vi "Positioner.vi"(8 "error in (no error)":errorcluster, 10 "Notifiers":T1, 11 "All Message Queue Cluster":T2) -> (0 "error out":errorcluster)   [LabVIEW 2013]
doc: "Ce VI est la partie visualisation du Positioner. Elle permet l'envoie d'ordre à cette appareil et affiche son état.\n- Connected : indique si l'appareil est connecté.\n- Position : indique la postion en mm du positioner.\n- Status : indique le status actuel du positioner. CAD s'il y a une erreur, ou s'il est en mouvement, etc ..."
uses:
  Lib QMH/AllMessageQueue Cluster.ctl
  Lib QMH/Message Cluster.ctl
  Lib Notifier/Notifier.ctl
  Pos UI data.ctl
  Pos Config.ctl
  FGV/Action Pos.ctl
  FGV/FGV Pos Data.ctl
  Lib IHM Control/Front Panel Status.ctl
  support/Status.vi
  Lib QMH/MessageQueues.lvlib
  Lib IHM Control/IHM Control.lvlib
  Lib Notifier/Notifier.lvlib
panel:
  out "Connected":bool
  out "Status":string
  out "Position (mm)":dbl format="%#_3g"
  # "Positionner"
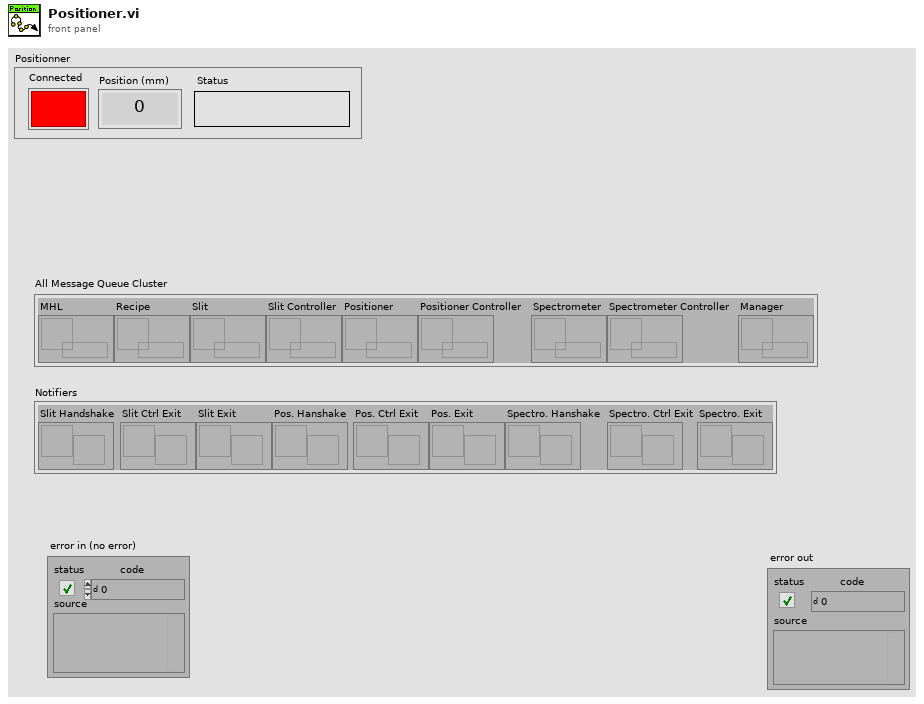
[diagram p1: front panel]
types:
  T1 = typedef "Notifier.lvlib/Notifier.ctl" = cluster{"Slit Handshake":refnum<notifier>, "Slit Ctrl Exit":refnum<notifier>, "Slit Exit":refnum<notifier>, "Pos. Hanshake":refnum<notifier>, "Pos. Ctrl Exit":refnum<notifier>, "Pos. Exit":refnum<notifier>, "Spectro. Hanshake":refnum<notifier>, "Spectro. Ctrl Exit":refnum<notifier>, "Spectro. Exit":refnum<notifier>}
  T2 = typedef "MessageQueues.lvlib/AllMessageQueue Cluster.ctl" = cluster{"MHL":refnum<queue>, "Recipe":refnum<queue>, "Slit":refnum<queue>, "Slit Controller":refnum<queue>, "Positioner":refnum<queue>, "Positioner Controller":refnum<queue>, "Spectrometer":refnum<queue>, "Spectrometer Controller":refnum<queue>, "Manager":refnum<queue>}
  T3 = typedef "Pos Config.ctl" = cluster{"VISA resource name":refnum<visa-resource-name>}
  T4 = typedef "Pos UI data.ctl" = cluster{"Connected":bool, "Status":string, "Position":dbl}
  T5 = typedef "Action Pos.ctl" = enum16{"Connect", "Initialize", "Set Velocity", "Get Velocity", "Move Rel", "Move Abs", "Position", "Status", "Abort", "Disconnect"}
  T6 = typedef "FGV Pos Data.ctl" = cluster{"Portnumber":i32, "Position":dbl, "Status":string, "Système ID":i32, "Connected axes":string[], "Velocity":dbl, "Stage names":string[], "Device ID out":i32}
  T7 = typedef "IHM Control.lvlib/Front Panel Status.ctl" = enum16{"Initialisation", "Enable Slit", "Enable Positionner", "Enable Spectrometer", "Disable Slit", "Disable Positionner", "Disable Spectrometer"}
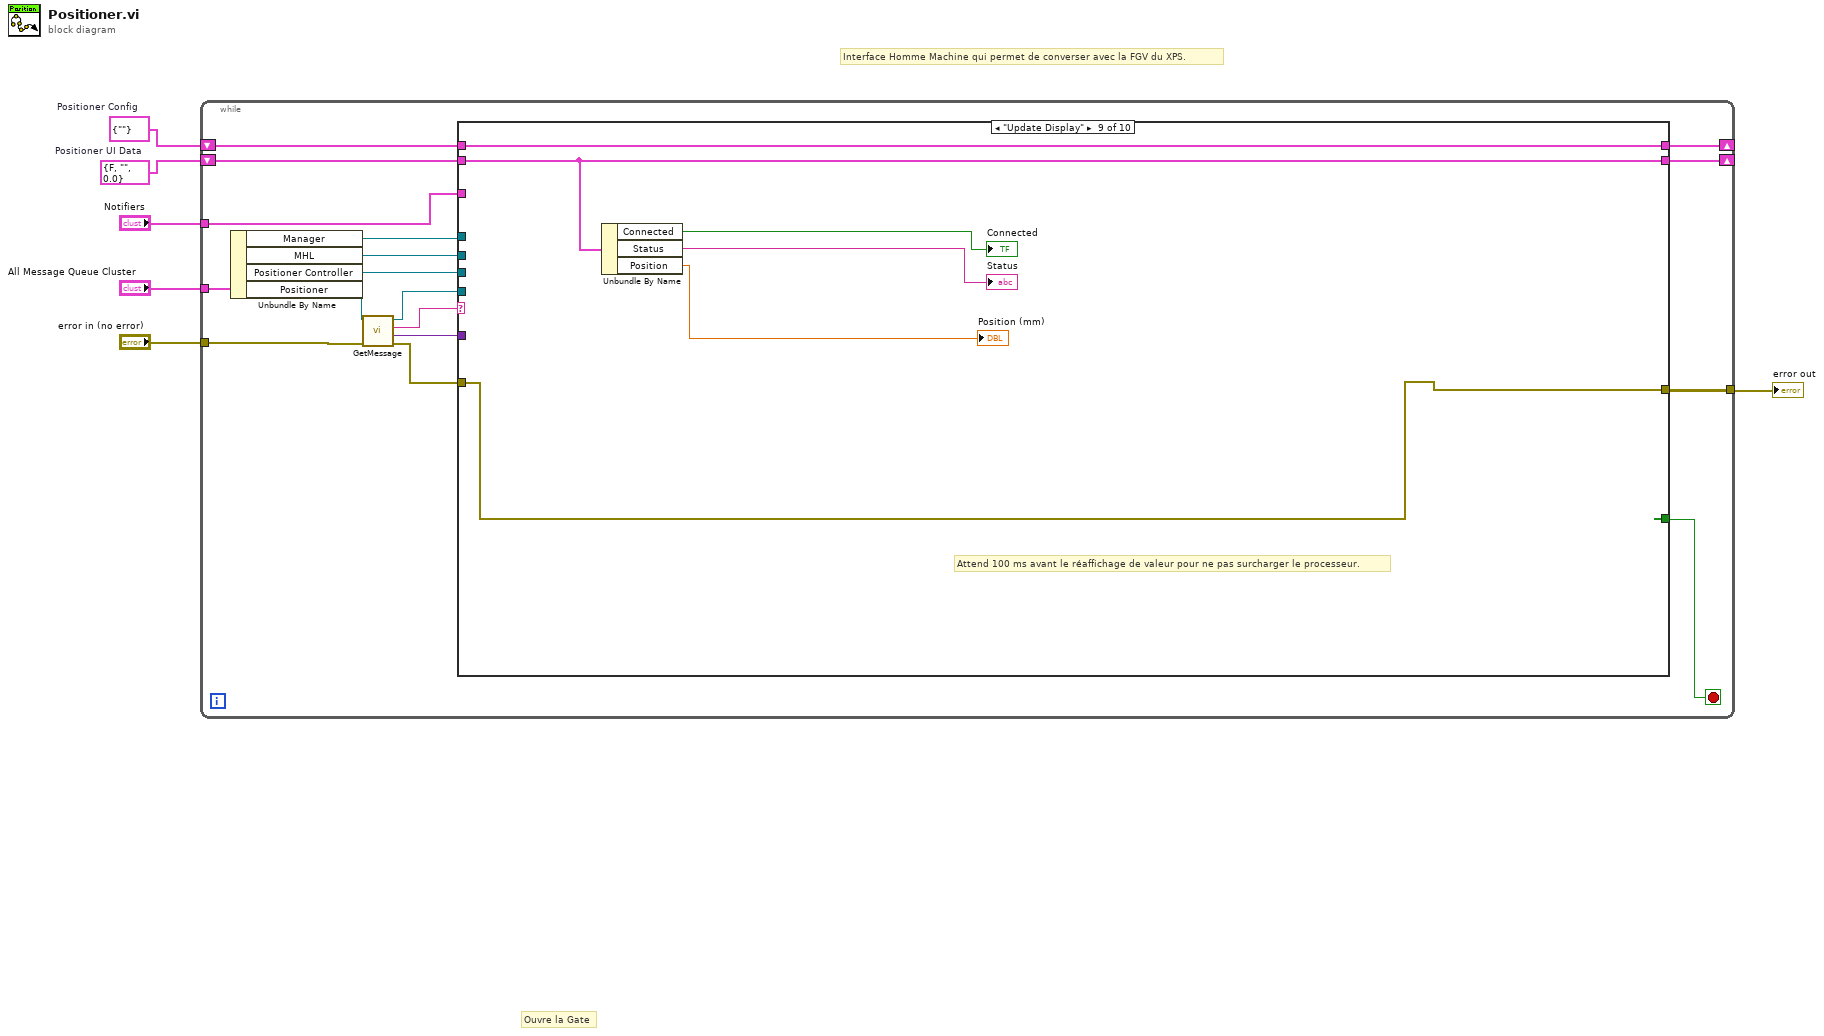
[diagram p0: block diagram]
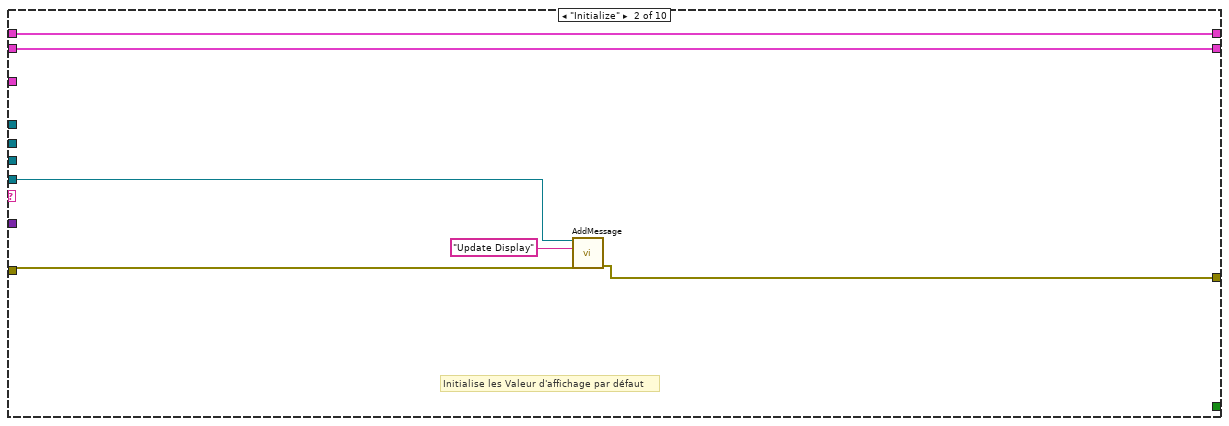
[diagram p3: hidden frame]
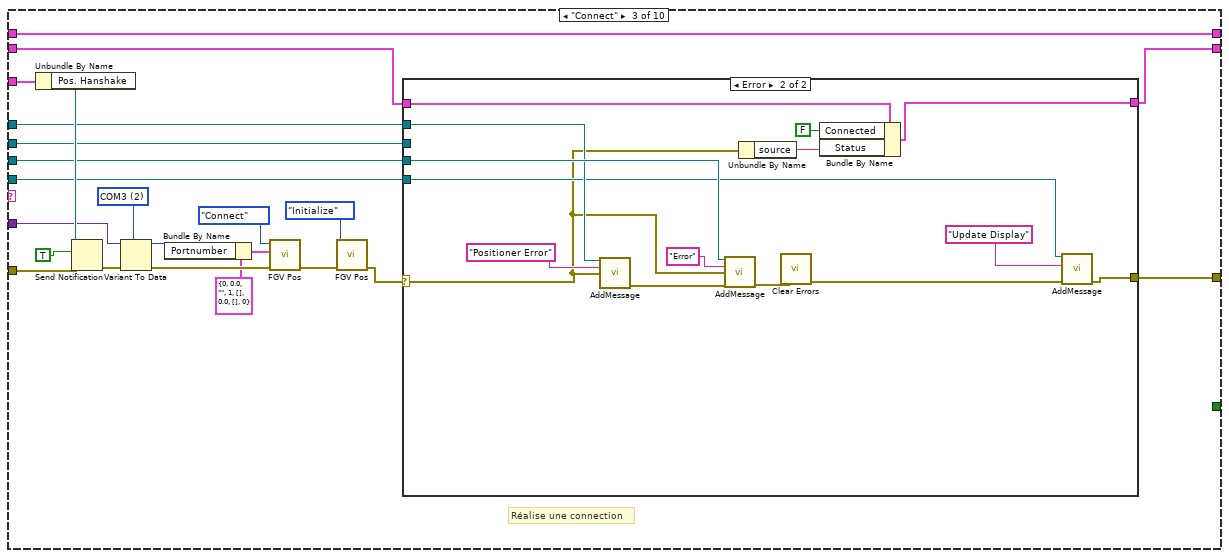
[diagram p4: hidden frame]
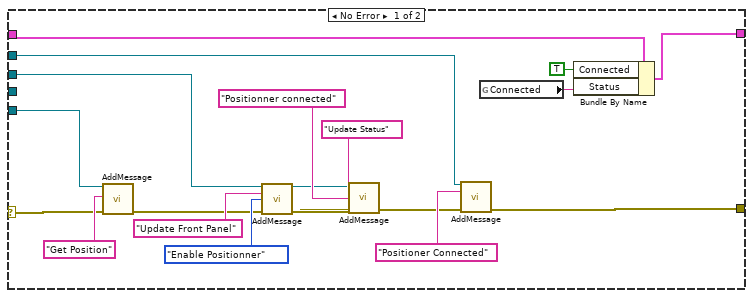
[diagram p5: hidden frame]
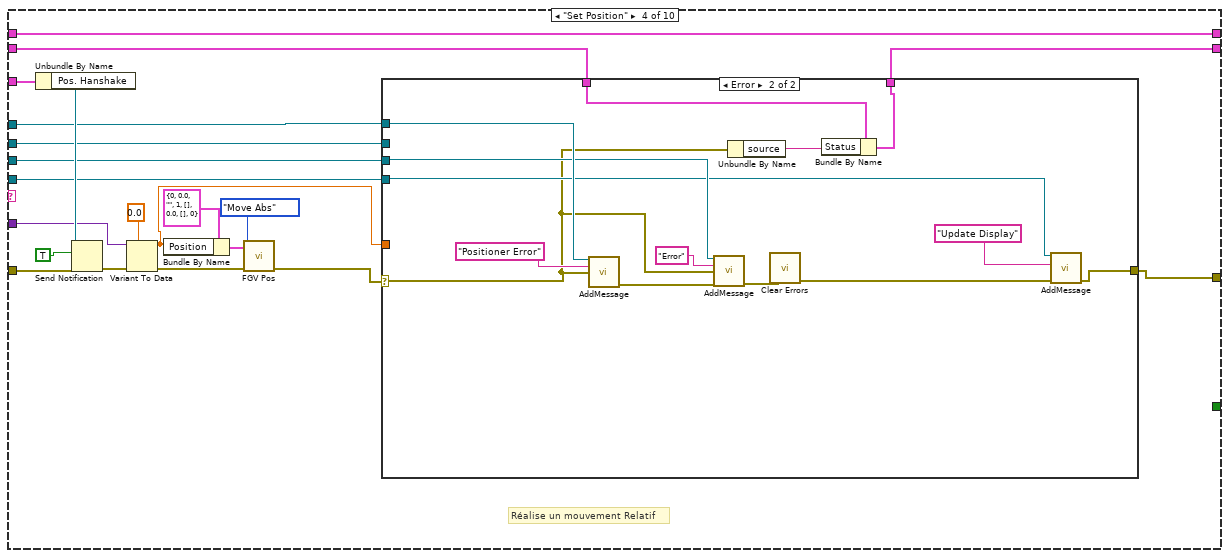
[diagram p6: hidden frame]
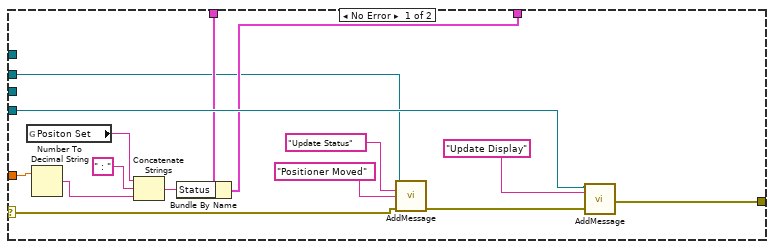
[diagram p7: hidden frame]
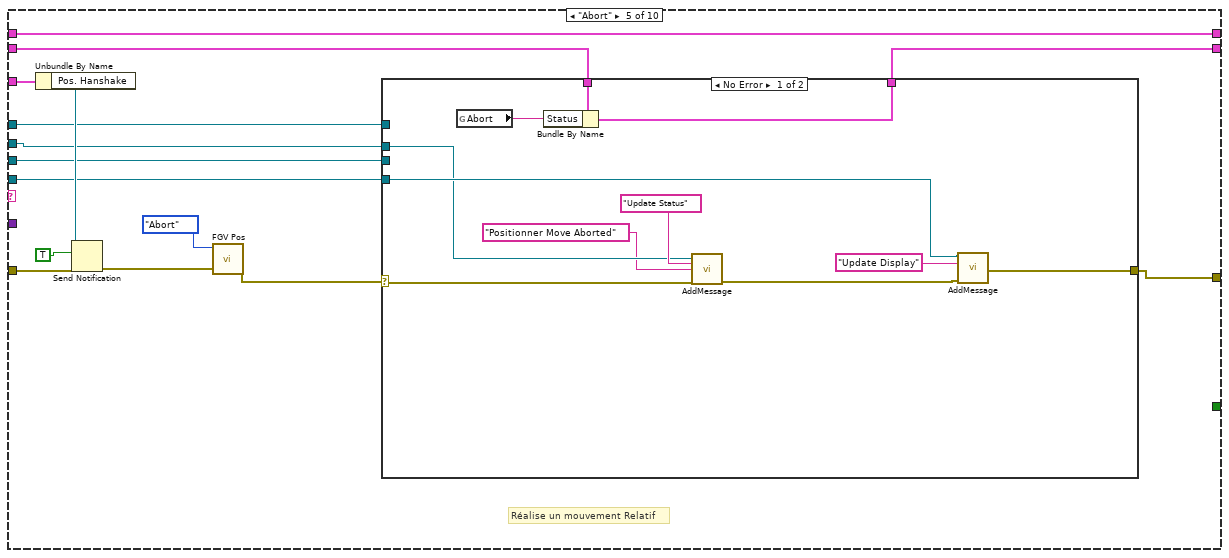
[diagram p8: hidden frame]
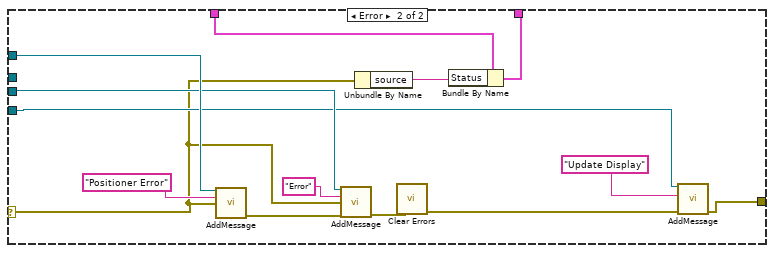
[diagram p9: hidden frame]
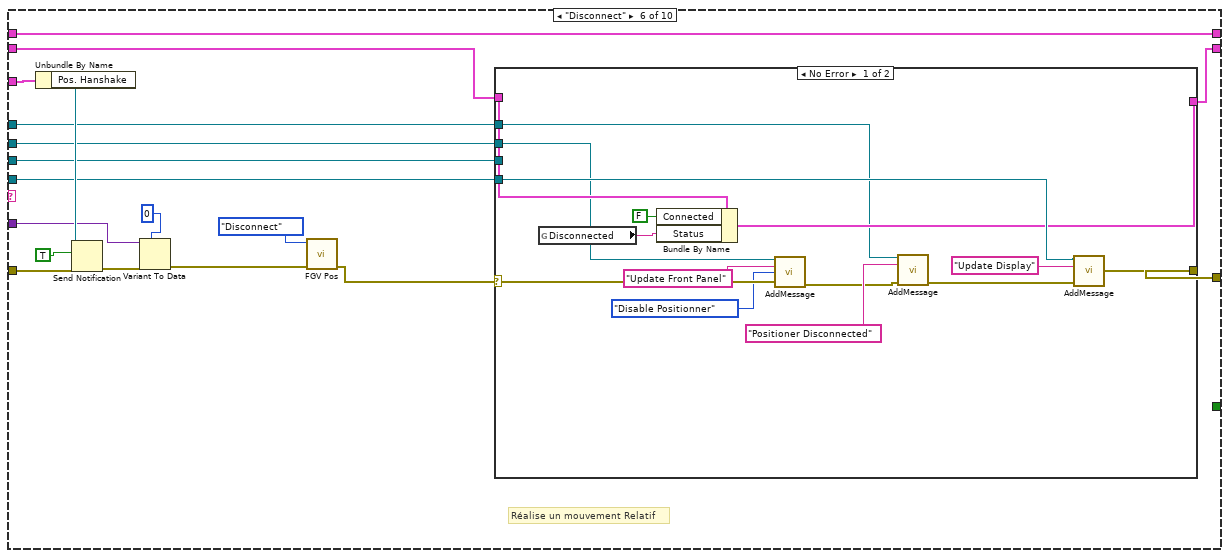
[diagram p10: hidden frame]
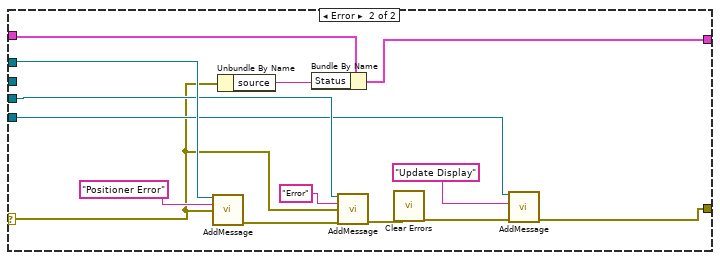
[diagram p11: hidden frame]
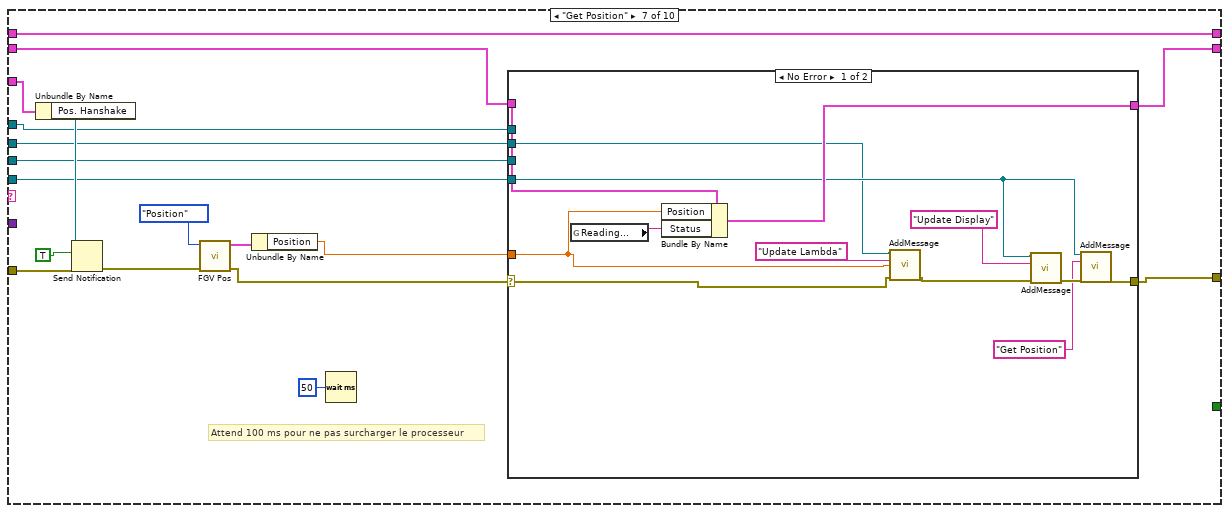
[diagram p12: hidden frame]
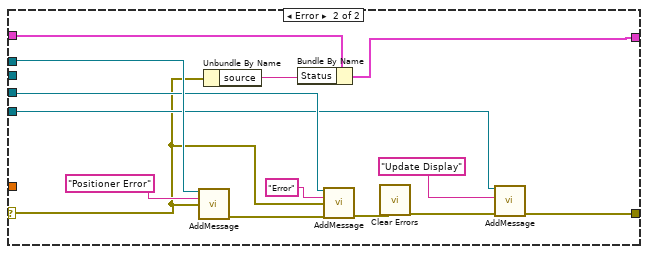
[diagram p13: hidden frame]
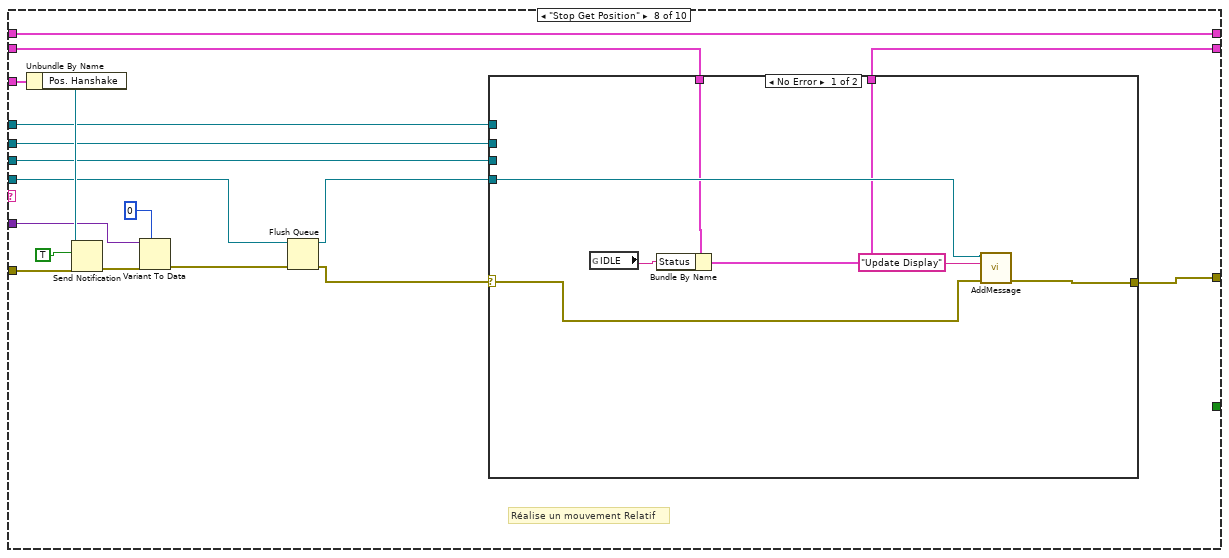
[diagram p14: hidden frame]
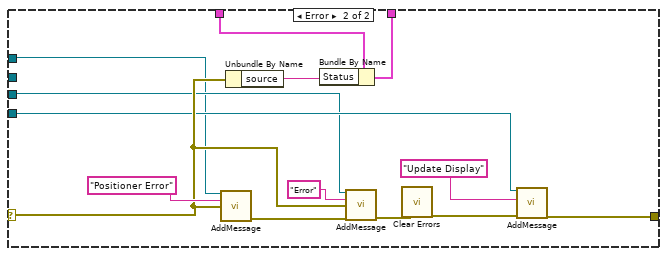
[diagram p15: hidden frame]
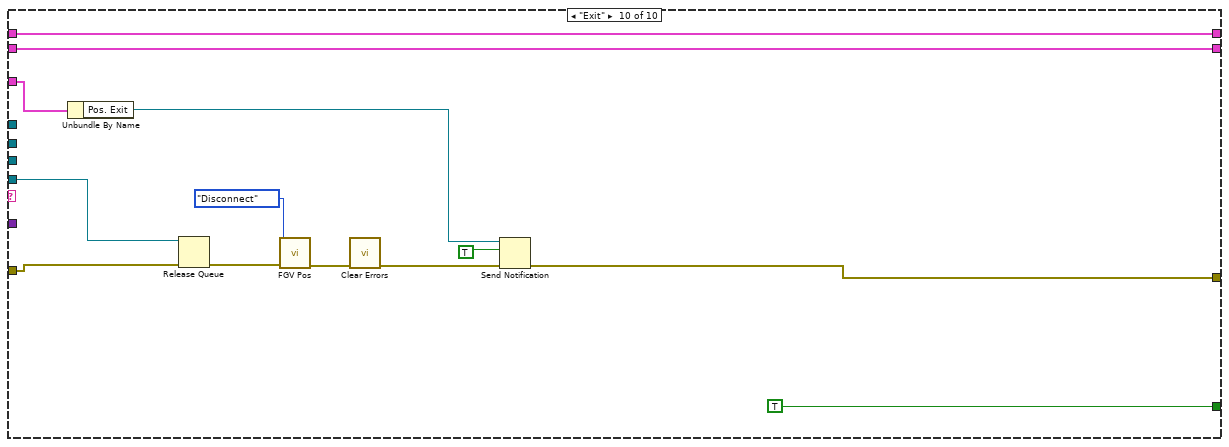
[diagram p16: hidden frame]
diagram:
  w1 = T3 {"VISA resource name"=""}  # Positioner Config
  w2 = T4 {"Connected"=FALSE, "Status"="", "Position"=0.0}  # Positioner UI Data
  # "Interface Homme Machine qui permet de converser avec la FGV du XPS."
  # "Ouvre la Gate"
  n1 = while {
    tunnel: "All Message Queue Cluster" -> [w21]
    tunnel: "Notifiers" -> [w18]
    tunnel: "error in (no error)" -> [w22]
    tunnel: [w10] -> w3
    shift-right: [w8] -> _
    shift-left: w1 -> [w20]
    shift-right: [w9] -> _
    shift-left: w2 -> [w19]
    stop <- w7 stop-if-true
    n2 = Unbundle By Name(w21) -> ("Manager"=w11:refnum<queue>, "MHL"=w12:refnum<queue>, "Positioner Controller"=w13:refnum<queue>, "Positioner"=w23:refnum<queue>)
    n3 = call "GetMessage.vi"("entrée d'erreur"=w22, "Message queue"=w23) -> ("sortie d'erreur"=w17:errorcluster, "Data"=w16:variant, "Message"=w15:string, "Dup Message Queue"=w14:refnum<queue>)  [unwired: 6 in]
    n4 = case shown="\"Update Display\"" w15 {
      tunnel: w18 -> [_ _ w53 w108 w152 w195 w242 w287 _ w328]
      tunnel: w14 -> [_ w27 w52 w107 w151 w194 w241 w275 _ w322]
      tunnel: w16 -> [_ _ w41 w97 _ w186 _ w279 _ _]
      tunnel: w17 -> [w26 w30 w46 w101 w145 w188 w236 w281 w315 w323]
      tunnel: [w26 w29 w51 w106 w150 w193 w240 w286 w315 w325] -> w10
      tunnel: w13 -> [_ _ w50 w105 w149 w192 w239 w285 _ _]
      tunnel: [_ _ _ _ _ _ _ _ _ TRUE] -> w7
      tunnel: w20 -> [w25 w32 w49 w104 w148 w191 w238 w284 w316 w324]
      tunnel: [w25 w32 w49 w104 w148 w191 w238 w284 w316 w324] -> w8
      tunnel: w19 -> [w24 w28 w48 w103 w147 w190 w233 w283 w314 w321]
      tunnel: [w24 w28 w47 w102 w146 w189 w237 w282 w314 w321] -> w9
      tunnel: w12 -> [_ _ w45 w100 w144 w184 w234 w272 _ _]
      tunnel: w11 -> [_ _ w44 w99 w143 w183 w227 w273 _ _]
      frame Default {
        # "ne fait rien si le message dépilé n'existe pas"
      }
      frame "Initialize" {
        # "Initialise les Valeur d'affichage par défaut"
        n5 = call "AddMessage.vi"("Message queue"=w27, "Message"="Update Display", "entrée d'erreur (pas d'erreur)"=w30) -> ("error out"=w29:errorcluster)  [unwired: 11 in, 1 out]
      }
      frame "Connect" {
        w42 = 2 items=["COM1", "COM2", "COM3", "COM4", "COM5", "COM6", "COM7", "COM8", "COM9", "COM10", "COM11", "COM12", "COM13", "COM14", "COM15", "COM16", "COM17", "COM18", "COM19", "COM20", "COM21", "COM22", "COM23", "COM24", "COM25", "COM26", "COM27", "COM28", "COM29", "COM30"] ("Portnumber")
        # "Réalise une connection"
        n6 = Unbundle By Name(w53) -> ("Pos. Hanshake"=w55:refnum<notifier>)
        n7 = Send Notification(notification=TRUE, notifier=w55, error in (no error)=w46) -> (error out=w43:errorcluster)  [unwired: 1 out]
        n8 = Variant To Data(error in=w43, type=w42, Variant=w41) -> (data=w37:i32, error out=w40:errorcluster)
        n9 = Bundle By Name(cluster=T6 {"Portnumber"=0, "Position"=0.0, "Status"="", "Système ID"=1, "Connected axes"=[], "Velocity"=0.0, "Stage names"=[], "Device ID out"=0} ("FGV Pos Data"), "Portnumber"=w37) -> (w36:T6)
        n10 = call "FGV Pos.vi"("error in (no error)"=w40, "FGV Pos Data In"=w36, "Action"=Action_Pos."Connect") -> ("error out"=w35:errorcluster)  [unwired: 7 in, 1 out]
        n11 = call "FGV Pos.vi"("error in (no error)"=w35, "Action"=Action_Pos."Initialize") -> ("error out"=w34:errorcluster)  [unwired: 8 in, 1 out]
        n12 = case shown="Error" w34 {
          selector: w34 -> [w59 w76]
          tunnel: w52 -> [w57 w81]
          tunnel: [w61 w85] -> w51
          tunnel: w50 -> [_ w84]
          tunnel: w48 -> [w74 w80]
          tunnel: [w73 w79] -> w47
          tunnel: w45 -> [w71 _]
          tunnel: w44 -> [w66 w82]
          frame No Error {
            n13 = call "AddMessage.vi"("Message queue"=w57, "Message"="Get Position", "entrée d'erreur (pas d'erreur)"=w59) -> ("error out"=w58:errorcluster)  [unwired: 11 in, 1 out]
            n14 = call "AddMessage.vi"("Message queue"=w71, "Message"="Update Front Panel", "Data"=Front_Panel_Status."Enable Positionner" ("Front Panel status"), "entrée d'erreur (pas d'erreur)"=w58) -> ("Dup Message queue"=w63:refnum<queue>, "error out"=w62:errorcluster)  [unwired: 10 in]
            n15 = call "AddMessage.vi"("Message queue"=w63, "Message"="Update Status", "Data"="Positionner connected" ("Message"), "entrée d'erreur (pas d'erreur)"=w62) -> ("error out"=w56:errorcluster)  [unwired: 10 in, 1 out]
            n16 = call "AddMessage.vi"("Message queue"=w66, "Message"="Positioner Connected", "entrée d'erreur (pas d'erreur)"=w56) -> ("error out"=w61:errorcluster)  [unwired: 11 in, 1 out]
            n17 = global read "Status.vi" "Connected"() -> (w67:string)
            n18 = Bundle By Name(cluster=w74, "Connected"=TRUE, "Status"=w67) -> (w73:T4)
          }
          frame Error {
            n19 = call "AddMessage.vi"("Message queue"=w82, "Message"="Positioner Error", "Data"=w76) -> ("error out"=w75:errorcluster)  [unwired: 11 in, 1 out]
            n20 = call "AddMessage.vi"("Message queue"=w84, "Message"="Error", "Data"=w76, "entrée d'erreur (pas d'erreur)"=w75) -> ("error out"=w88:errorcluster)  [unwired: 10 in, 1 out]
            n21 = Unbundle By Name(w76) -> ("source"=w77:string)
            n22 = call <vilib>:"Clear Errors.vi"("error in (no error)"=w88) -> ("error out"=w86:errorcluster)  [unwired: 6 in]
            n23 = Bundle By Name(cluster=w80, "Connected"=FALSE, "Status"=w77) -> (w79:T4)
            n24 = call "AddMessage.vi"("Message queue"=w81, "Message"="Update Display", "entrée d'erreur (pas d'erreur)"=w86) -> ("error out"=w85:errorcluster)  [unwired: 11 in, 1 out]
          }
        }
      }
      frame "Set Position" {
        # "Réalise un mouvement Relatif"
        n25 = Unbundle By Name(w108) -> ("Pos. Hanshake"=w110:refnum<notifier>)
        n26 = Send Notification(notification=TRUE, notifier=w110, error in (no error)=w101) -> (error out=w98:errorcluster)  [unwired: 1 out]
        n27 = Variant To Data(error in=w98, type=0.0, Variant=w97) -> (data=w90:dbl, error out=w95:errorcluster)
        n28 = Bundle By Name(cluster=T6 {"Portnumber"=0, "Position"=0.0, "Status"="", "Système ID"=1, "Connected axes"=[], "Velocity"=0.0, "Stage names"=[], "Device ID out"=0} ("FGV Pos Data"), "Position"=w90) -> (w92:T6)
        n29 = call "FGV Pos.vi"("error in (no error)"=w95, "FGV Pos Data In"=w92, "Action"=Action_Pos."Move Abs") -> ("error out"=w94:errorcluster)  [unwired: 7 in, 1 out]
        n30 = case shown="Error" w94 {
          selector: w94 -> [w113 w127]
          tunnel: w107 -> [w125 w128]
          tunnel: [w123 w126] -> w106
          tunnel: w105 -> [_ w129]
          tunnel: w103 -> [w122 w132]
          tunnel: [w121 w131] -> w102
          tunnel: w100 -> [w111 _]
          tunnel: w99 -> [_ w130]
          tunnel: w90 -> [w117 _]
          frame No Error {
            n31 = global read "Status.vi" "Positon Set"() -> (w120:string)
            n32 = Number To Decimal String(number=w117) -> (decimal integer string=w116:string)  [unwired: 1 in]
            n33 = Concatenate Strings(w120, " : " ("string"), w116) -> (w119:string)
            n34 = Bundle By Name(cluster=w122, "Status"=w119) -> (w121:T4)
            n35 = call "AddMessage.vi"("Message queue"=w111, "Message"="Update Status", "Data"="Positioner Moved" ("Message"), "entrée d'erreur (pas d'erreur)"=w113) -> ("error out"=w112:errorcluster)  [unwired: 10 in, 1 out]
            n36 = call "AddMessage.vi"("Message queue"=w125, "Message"="Update Display", "entrée d'erreur (pas d'erreur)"=w112) -> ("error out"=w123:errorcluster)  [unwired: 11 in, 1 out]
          }
          frame Error {
            n37 = call "AddMessage.vi"("Message queue"=w130, "Message"="Positioner Error", "Data"=w127) -> ("error out"=w133:errorcluster)  [unwired: 11 in, 1 out]
            n38 = call "AddMessage.vi"("Message queue"=w129, "Message"="Error", "Data"=w127, "entrée d'erreur (pas d'erreur)"=w133) -> ("error out"=w138:errorcluster)  [unwired: 10 in, 1 out]
            n39 = Unbundle By Name(w127) -> ("source"=w134:string)
            n40 = call <vilib>:"Clear Errors.vi"("error in (no error)"=w138) -> ("error out"=w136:errorcluster)  [unwired: 6 in]
            n41 = Bundle By Name(cluster=w132, "Status"=w134) -> (w131:T4)
            n42 = call "AddMessage.vi"("Message queue"=w128, "Message"="Update Display", "entrée d'erreur (pas d'erreur)"=w136) -> ("error out"=w126:errorcluster)  [unwired: 11 in, 1 out]
          }
        }
      }
      frame "Abort" {
        # "Réalise un mouvement Relatif"
        n43 = Unbundle By Name(w152) -> ("Pos. Hanshake"=w154:refnum<notifier>)
        n44 = Send Notification(notification=TRUE, notifier=w154, error in (no error)=w145) -> (error out=w142:errorcluster)  [unwired: 1 out]
        n45 = call "FGV Pos.vi"("error in (no error)"=w142, "Action"=Action_Pos."Abort") -> ("error out"=w141:errorcluster)  [unwired: 8 in, 1 out]
        n46 = case shown="No Error" w141 {
          selector: w141 -> [w158 w169]
          tunnel: w151 -> [w165 w170]
          tunnel: [w163 w166] -> w150
          tunnel: w149 -> [_ w171]
          tunnel: w147 -> [w162 w168]
          tunnel: [w161 w167] -> w146
          tunnel: w144 -> [w157 _]
          tunnel: w143 -> [_ w172]
          frame No Error {
            n47 = global read "Status.vi" "Abort"() -> (w160:string)
            n48 = Bundle By Name(cluster=w162, "Status"=w160) -> (w161:T4)
            n49 = call "AddMessage.vi"("Message queue"=w157, "Message"="Update Status", "Data"="Positionner Move Aborted" ("Message"), "entrée d'erreur (pas d'erreur)"=w158) -> ("error out"=w155:errorcluster)  [unwired: 10 in, 1 out]
            n50 = call "AddMessage.vi"("Message queue"=w165, "Message"="Update Display", "entrée d'erreur (pas d'erreur)"=w155) -> ("error out"=w163:errorcluster)  [unwired: 11 in, 1 out]
          }
          frame Error {
            n51 = call "AddMessage.vi"("Message queue"=w172, "Message"="Positioner Error", "Data"=w169) -> ("error out"=w173:errorcluster)  [unwired: 11 in, 1 out]
            n52 = call "AddMessage.vi"("Message queue"=w171, "Message"="Error", "Data"=w169, "entrée d'erreur (pas d'erreur)"=w173) -> ("error out"=w178:errorcluster)  [unwired: 10 in, 1 out]
            n53 = Unbundle By Name(w169) -> ("source"=w174:string)
            n54 = call <vilib>:"Clear Errors.vi"("error in (no error)"=w178) -> ("error out"=w176:errorcluster)  [unwired: 6 in]
            n55 = Bundle By Name(cluster=w168, "Status"=w174) -> (w167:T4)
            n56 = call "AddMessage.vi"("Message queue"=w170, "Message"="Update Display", "entrée d'erreur (pas d'erreur)"=w176) -> ("error out"=w166:errorcluster)  [unwired: 11 in, 1 out]
          }
        }
      }
      frame "Disconnect" {
        # "Réalise un mouvement Relatif"
        n57 = Unbundle By Name(w195) -> ("Pos. Hanshake"=w197:refnum<notifier>)
        n58 = Send Notification(notification=TRUE, notifier=w197, error in (no error)=w188) -> (error out=w187:errorcluster)  [unwired: 1 out]
        n59 = Variant To Data(error in=w187, type=0, Variant=w186) -> (error out=w182:errorcluster)  [unwired: 1 out]
        n60 = call "FGV Pos.vi"("error in (no error)"=w182, "Action"=Action_Pos."Disconnect") -> ("error out"=w181:errorcluster)  [unwired: 8 in, 1 out]
        n61 = case shown="No Error" w181 {
          selector: w181 -> [w206 w216]
          tunnel: w194 -> [w212 w217]
          tunnel: [w210 w215] -> w193
          tunnel: w192 -> [_ w218]
          tunnel: w190 -> [w209 w214]
          tunnel: [w208 w213] -> w189
          tunnel: w184 -> [w205 _]
          tunnel: w183 -> [w199 w219]
          frame No Error {
            n62 = global read "Status.vi" "Disconnected"() -> (w198:string)
            n63 = Bundle By Name(cluster=w209, "Connected"=FALSE, "Status"=w198) -> (w208:T4)
            n64 = call "AddMessage.vi"("Message queue"=w205, "Message"="Update Front Panel", "Data"=Front_Panel_Status."Disable Positionner" ("Front Panel status"), "entrée d'erreur (pas d'erreur)"=w206) -> ("error out"=w201:errorcluster)  [unwired: 10 in, 1 out]
            n65 = call "AddMessage.vi"("Message queue"=w199, "Message"="Positioner Disconnected", "entrée d'erreur (pas d'erreur)"=w201) -> ("error out"=w200:errorcluster)  [unwired: 11 in, 1 out]
            n66 = call "AddMessage.vi"("Message queue"=w212, "Message"="Update Display", "entrée d'erreur (pas d'erreur)"=w200) -> ("error out"=w210:errorcluster)  [unwired: 11 in, 1 out]
          }
          frame Error {
            n67 = call "AddMessage.vi"("Message queue"=w219, "Message"="Positioner Error", "Data"=w216) -> ("error out"=w220:errorcluster)  [unwired: 11 in, 1 out]
            n68 = Unbundle By Name(w216) -> ("source"=w221:string)
            n69 = Bundle By Name(cluster=w214, "Status"=w221) -> (w213:T4)
            n70 = call "AddMessage.vi"("Message queue"=w218, "Message"="Error", "Data"=w216, "entrée d'erreur (pas d'erreur)"=w220) -> ("error out"=w225:errorcluster)  [unwired: 10 in, 1 out]
            n71 = call <vilib>:"Clear Errors.vi"("error in (no error)"=w225) -> ("error out"=w223:errorcluster)  [unwired: 6 in]
            n72 = call "AddMessage.vi"("Message queue"=w217, "Message"="Update Display", "entrée d'erreur (pas d'erreur)"=w223) -> ("error out"=w215:errorcluster)  [unwired: 11 in, 1 out]
          }
        }
      }
      frame "Get Position" {
        # "Attend 100 ms pour ne pas surcharger le processeur"
        n73 = Unbundle By Name(w242) -> ("Pos. Hanshake"=w244:refnum<notifier>)
        n74 = Send Notification(notification=TRUE, notifier=w244, error in (no error)=w236) -> (error out=w232:errorcluster)  [unwired: 1 out]
        n75 = call "FGV Pos.vi"("error in (no error)"=w232, "Action"=Action_Pos."Position") -> ("error out"=w230:errorcluster, "FGV Pos Data Out"=w229:T6)  [unwired: 8 in]
        n76 = Unbundle By Name(w229) -> ("Position"=w228:dbl)
        n77 = Wait (ms)(milliseconds to wait=u32 50) -> ()  [unwired: 1 out]
        n78 = case shown="No Error" w230 {
          selector: w230 -> [w248 w258]
          tunnel: w241 -> [w252 w259]
          tunnel: [w253 w264] -> w240
          tunnel: w239 -> [_ w260]
          tunnel: w233 -> [w256 w262]
          tunnel: [w255 w263] -> w237
          tunnel: w234 -> [w246 _]
          tunnel: w228 -> [w245 _]
          tunnel: w227 -> [_ w261]
          frame No Error {
            n79 = global read "Status.vi" "Reading..."() -> (w250:string)
            n80 = Bundle By Name(cluster=w256, "Position"=w245, "Status"=w250) -> (w255:T4)
            n81 = call "AddMessage.vi"("Message queue"=w246, "Message"="Update Lambda", "Data"=w245, "entrée d'erreur (pas d'erreur)"=w248) -> ("error out"=w247:errorcluster)  [unwired: 10 in, 1 out]
            n82 = call "AddMessage.vi"("Message queue"=w252, "Message"="Update Display", "entrée d'erreur (pas d'erreur)"=w247) -> ("error out"=w254:errorcluster)  [unwired: 11 in, 1 out]
            n83 = call "AddMessage.vi"("Message queue"=w252, "Message"="Get Position", "entrée d'erreur (pas d'erreur)"=w254) -> ("error out"=w253:errorcluster)  [unwired: 11 in, 1 out]
          }
          frame Error {
            n84 = call "AddMessage.vi"("Message queue"=w261, "Message"="Positioner Error", "Data"=w258) -> ("error out"=w265:errorcluster)  [unwired: 11 in, 1 out]
            n85 = Unbundle By Name(w258) -> ("source"=w266:string)
            n86 = Bundle By Name(cluster=w262, "Status"=w266) -> (w263:T4)
            n87 = call "AddMessage.vi"("Message queue"=w260, "Message"="Error", "Data"=w258, "entrée d'erreur (pas d'erreur)"=w265) -> ("error out"=w270:errorcluster)  [unwired: 10 in, 1 out]
            n88 = call <vilib>:"Clear Errors.vi"("error in (no error)"=w270) -> ("error out"=w268:errorcluster)  [unwired: 6 in]
            n89 = call "AddMessage.vi"("Message queue"=w259, "Message"="Update Display", "entrée d'erreur (pas d'erreur)"=w268) -> ("error out"=w264:errorcluster)  [unwired: 11 in, 1 out]
          }
        }
      }
      frame "Stop Get Position" {
        # "Réalise un mouvement Relatif"
        n90 = Unbundle By Name(w287) -> ("Pos. Hanshake"=w289:refnum<notifier>)
        n91 = Send Notification(notification=TRUE, notifier=w289, error in (no error)=w281) -> (error out=w280:errorcluster)  [unwired: 1 out]
        n92 = Variant To Data(error in=w280, type=0, Variant=w279) -> (error out=w277:errorcluster)  [unwired: 1 out]
        n93 = Flush Queue(queue=w275, error in (no error)=w277) -> (queue out=w274:refnum<queue>, error out=w276:errorcluster)  [unwired: 1 out]
        n94 = case shown="No Error" w276 {
          selector: w276 -> [w293 w303]
          tunnel: w274 -> [w296 w302]
          tunnel: [w294 w299] -> w286
          tunnel: w285 -> [_ w301]
          tunnel: w283 -> [w292 w298]
          tunnel: [w291 w297] -> w282
          tunnel: w273 -> [_ w300]
          tunnel: w272 -> [_ _]
          frame No Error {
            n95 = global read "Status.vi" "IDLE"() -> (w290:string)
            n96 = Bundle By Name(cluster=w292, "Status"=w290) -> (w291:T4)
            n97 = call "AddMessage.vi"("Message queue"=w296, "Message"="Update Display", "entrée d'erreur (pas d'erreur)"=w293) -> ("error out"=w294:errorcluster)  [unwired: 11 in, 1 out]
          }
          frame Error {
            n98 = call "AddMessage.vi"("Message queue"=w300, "Message"="Positioner Error", "Data"=w303) -> ("error out"=w304:errorcluster)  [unwired: 11 in, 1 out]
            n99 = Unbundle By Name(w303) -> ("source"=w305:string)
            n100 = Bundle By Name(cluster=w298, "Status"=w305) -> (w297:T4)
            n101 = call "AddMessage.vi"("Message queue"=w301, "Message"="Error", "Data"=w303, "entrée d'erreur (pas d'erreur)"=w304) -> ("error out"=w309:errorcluster)  [unwired: 10 in, 1 out]
            n102 = call <vilib>:"Clear Errors.vi"("error in (no error)"=w309) -> ("error out"=w307:errorcluster)  [unwired: 6 in]
            n103 = call "AddMessage.vi"("Message queue"=w302, "Message"="Update Display", "entrée d'erreur (pas d'erreur)"=w307) -> ("error out"=w299:errorcluster)  [unwired: 11 in, 1 out]
          }
        }
      }
      frame "Update Display" {
        # "Attend 100 ms avant le réaffichage de valeur pour ne pas surcharger le processeur."
        n104 = Unbundle By Name(w314) -> ("Connected"=→"Connected":bool, "Status"=→"Status":string, "Position"=→"Position (mm)":dbl)
      }
      frame "Exit" {
        n105 = Unbundle By Name(w328) -> ("Pos. Exit"=w327:refnum<notifier>)
        n106 = Release Queue(queue=w322, error in (no error)=w323) -> (error out=w320:errorcluster)  [unwired: 1 in, 2 out]
        n107 = call "FGV Pos.vi"("error in (no error)"=w320, "Action"=Action_Pos."Disconnect") -> ("error out"=w319:errorcluster)  [unwired: 8 in, 1 out]
        n108 = call <vilib>:"Clear Errors.vi"("error in (no error)"=w319) -> ("error out"=w318:errorcluster)  [unwired: 6 in]
        n109 = Send Notification(notification=TRUE, notifier=w327, error in (no error)=w318) -> (error out=w325:errorcluster)  [unwired: 1 out]
      }
    }
  }
  "error out" <- w3
